vi "Advanced Multi-Point Benchmark.vi"() -> ()   [LabVIEW 2011]
panel:
  in  "Multi Point Acquisition:Trigger Count":i32
  in  "Trigger:Trigger Source":i32(ring)=1 items=["NIDMM_VAL_IMMEDIATE"=1, "NIDMM_VAL_EXTERNAL"=2, "NIDMM_VAL_SOFTWARE_TRIG"=3, "NIDMM_VAL_TTL0"=111, "NIDMM_VAL_TTL1"=112, "NIDMM_VAL_TTL2"=113, "NIDMM_VAL_TTL3"=114, "NIDMM_VAL_TTL4"=115, "NIDMM_VAL_TTL5"=116, "NIDMM_VAL_TTL6"=117, "NIDMM_VAL_TTL7"=118, "NIDMM_VAL_PXI_STAR"=131, "NIDMM_VAL_LBR_TRIG_1"=1004, "NIDMM_VAL_AUX_TRIG_1"=1001]
  in  "Multi Point Acquisition:Sample Count":i32
  in  "Multi Point Acquisition:Sample Trigger":i32(ring)=1 items=["NIDMM_VAL_IMMEDIATE"=1, "NIDMM_VAL_INTERVAL"=10, "NIDMM_VAL_EXTERNAL"=2, "NIDMM_VAL_SOFTWARE_TRIG"=3, "NIDMM_VAL_TTL0"=111, "NIDMM_VAL_TTL1"=112, "NIDMM_VAL_TTL2"=113, "NIDMM_VAL_TTL3"=114, "NIDMM_VAL_TTL4"=115, "NIDMM_VAL_TTL5"=116, "NIDMM_VAL_TTL6"=117, "NIDMM_VAL_TTL7"=118, "NIDMM_VAL_PXI_STAR"=131, "NIDMM_VAL_LBR_TRIG_1"=1004, "NIDMM_VAL_AUX_TRIG_1"=1001]
  in  "Configuration:Measurement Options:DC Noise Rejection":i32(ring)=2 items=["Auto"=-1, "Normal"=0, "Second_Order"=1, "High_Order"=2]
  in  "Configuration:Advanced:Settle Time":dbl=0.001
  in  "Configuration:Advanced:Aperture Time":dbl=0.1
  in  "Configuration:Advanced:Aperture Time Units":i32(ring) items=["NIDMM_VAL_SECONDS", "NIDMM_VAL_POWER_LINE_CYCLES"]
  in  "Configuration:Function":i32(ring)=1 items=["NIDMM_VAL_DC_VOLTS"=1, "NIDMM_VAL_AC_VOLTS"=2, "NIDMM_VAL_DC_CURRENT"=3, "NIDMM_VAL_AC_CURRENT"=4, "NIDMM_VAL_2_WIRE_RES"=5, "NIDMM_VAL_4_WIRE_RES"=101, "NIDMM_VAL_FREQ"=104, "NIDMM_VAL_PERIOD"=105, "NIDMM_VAL_AC_VOLTS_DC_COUPLED"=1001, "NIDMM_VAL_DIODE"=1002, "NIDMM_VAL_CAPACITANCE"=1005, "NIDMM_VAL_INDUCTANCE"=1006, "NIDMM_VAL_WAVEFORM_VOLTAGE"=1003, "NIDMM_VAL_WAVEFORM_CURRENT"=1004]
  in  "Configuration:Range":dbl=10.0
  in  "Configuration:Measurement Options:ADC Calibration":i32(ring)=1 items=["Auto"=-1, "Off"=0, "On"=1]
  in  "Configuration:Measurement Options:Auto Zero":i32(ring)=1 items=["Auto"=-1, "Off"=0, "On"=1, "Once"=2]
  out "Measurement Period (seconds)":dbl format="%.4f"
  in  "Instrument Descriptor":refnum<k15>="DMM"
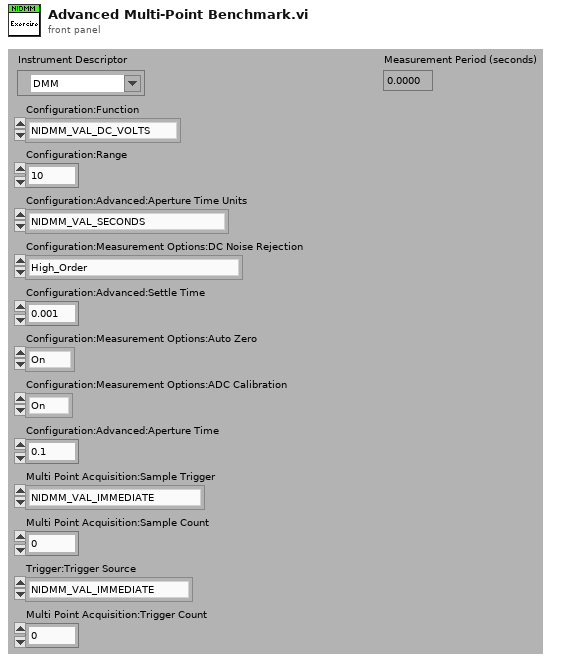
[diagram p1: front panel]
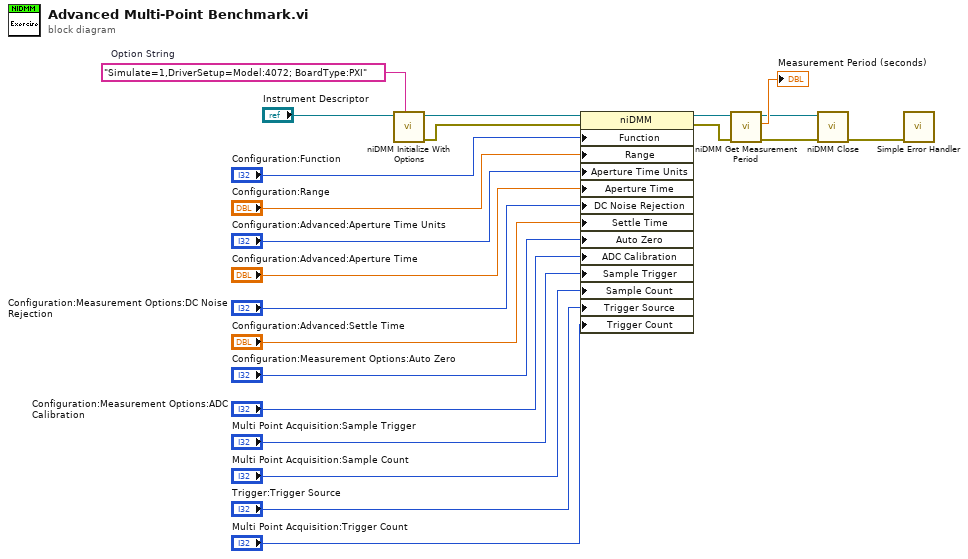
[diagram p0: block diagram]
diagram:
  w17 = "Simulate=1,DriverSetup=Model:4072; BoardType:PXI"  # Option String
  n1 = call <instrlib>:"niDMM Initialize With Options.vi"("Option String"=w17, "Instrument Descriptor"="Instrument Descriptor") -> ("error out"=w6:errorcluster, "instrument handle out"=w16:refnum<k15>)  [unwired: 8 in]
  n2 = property class="niDMM"(reference=w16, error in=w6, "Function"="Configuration:Function", "Range"="Configuration:Range", "Aperture Time Units"="Configuration:Advanced:Aperture Time Units", "Aperture Time"="Configuration:Advanced:Aperture Time", "DC Noise Rejection"="Configuration:Measurement Options:DC Noise Rejection", "Settle Time"="Configuration:Advanced:Settle Time", "Auto Zero"="Configuration:Measurement Options:Auto Zero", "ADC Calibration"="Configuration:Measurement Options:ADC Calibration", "Sample Trigger"="Multi Point Acquisition:Sample Trigger", "Sample Count"="Multi Point Acquisition:Sample Count", "Trigger Source"="Trigger:Trigger Source", "Trigger Count"="Multi Point Acquisition:Trigger Count") -> (reference out=w7:refnum<k15>, error out=w1:errorcluster)
  n3 = call <instrlib>:"niDMM Get Measurement Period.vi"("error in (no error)"=w1, "instrument handle"=w7) -> ("error out"=w20:errorcluster, "Measurement Period (seconds)"=→"Measurement Period (seconds)":dbl, "instrument handle out"=w19:refnum<k15>)  [unwired: 7 in]
  n4 = call <instrlib>:"niDMM Close.vi"("error in (no error)"=w20, "instrument handle"=w19) -> ("error out"=w18:errorcluster)  [unwired: 9 in]
  n5 = call <vilib>:"Simple Error Handler.vi"("error in (no error)"=w18) -> ()  [unwired: 4 in, 5 out]
